vi "python2.vi"() -> ()   [LabVIEW 2011]
panel:
  out "Return Code":i64
  out "Error":string
  out "Output":string
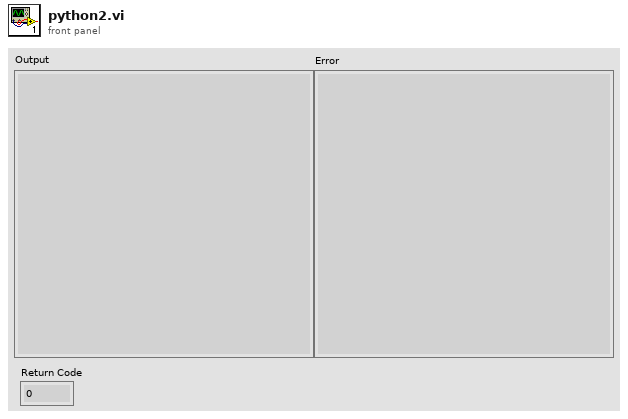
[diagram p1: front panel]
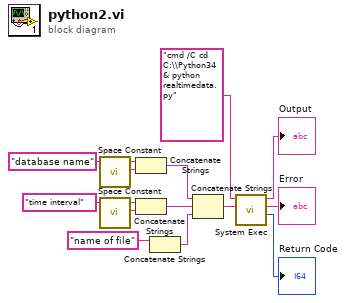
[diagram p0: block diagram]
diagram:
  n1 = call <vilib>:"Space Constant.vi"() -> ("String"=w8:string)
  n2 = call <vilib>:"Space Constant.vi"() -> ("String"=w6:string)
  n3 = Concatenate Strings("database name", w8) -> (w4:string)
  n4 = Concatenate Strings("time interval", w6) -> (w3:string)
  n5 = Concatenate Strings("name of file") -> (w2:string)  [unwired: 1 in]
  n6 = Concatenate Strings(w4, w3, w2) -> (w1:string)
  n7 = call <vilib>:"System Exec.vi"("standard input"=w1, "command line"="cmd /C cd C:\\Python34  & python realtimedata.py") -> ("return code"=→"Return Code":i32, "standard error"=→"Error":string, "standard output"=→"Output":string)  [unwired: 6 in, 1 out]
